vi "Template_Regular_NoReturn.vi"(8 "Error In":errorcluster, 11 "OpaqueStruct In":refnum<class "TEMPLATE_OpaqueStruct.lvclass">) -> (0 "Error Out":errorcluster, 3 "OpaqueStruct Out":refnum<class "TEMPLATE_OpaqueStruct.lvclass">)   [LabVIEW 2013, in "Template.lvlib" / "TEMPLATE_OpaqueStruct.lvclass"]
uses:
  TEMPLATE_OpaqueStruct.lvclass
  TEMPLATE_OpaqueStruct.lvclass/TEMPLATE_OpaqueStruct.ctl
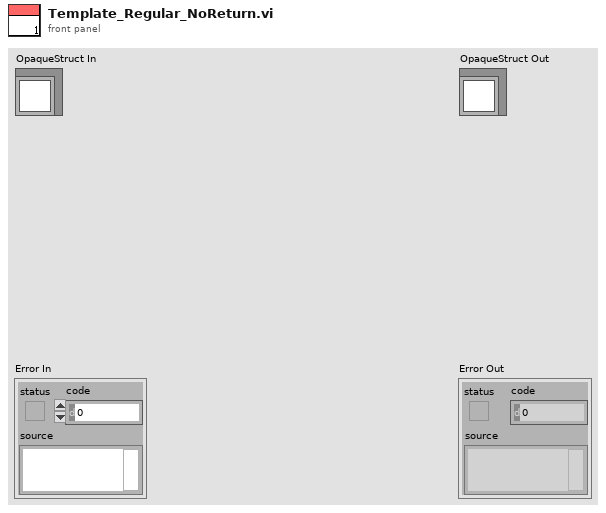
[diagram p1: front panel]
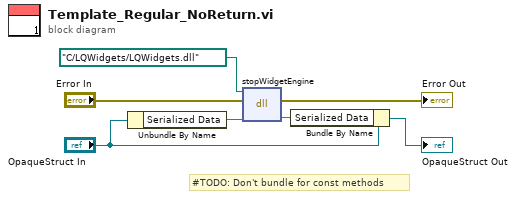
[diagram p0: block diagram]
diagram:
  # "#TODO: Don't bundle for const methods"
  n1 = Unbundle By Name("OpaqueStruct In") -> ("Serialized Data"=w4:string)
  n2 = dll-call lib="?" fn="stopWidgetEngine"(path in=path "C:/LQWidgets/LQWidgets.dll", error in="Error In", "obj"=w4) -> (error out=→"Error Out":errorcluster, "obj"=w3:string)  [unwired: 2 in, 1 out]
  n3 = Bundle By Name(cluster="OpaqueStruct In", "Serialized Data"=w3) -> (→"OpaqueStruct Out":refnum<class "TEMPLATE_OpaqueStruct.lvclass">)
